vi "AppendObjectNameIfError.vi"(8 "error in (no error)":errorcluster, 10 "GObj Refnum":refnum<vi>, 11 "Control Layout in":refnum<class "Control Layout.lvclass">) -> (0 "error out":errorcluster, 3 "Control Layout out":refnum<class "Control Layout.lvclass">)   [LabVIEW 2010, in "NI_SE_Front Panel Layout.lvlib" / "Control Layout.lvclass"]
uses:
  Control Layout.lvclass
  Object Layout/Object Layout.lvclass
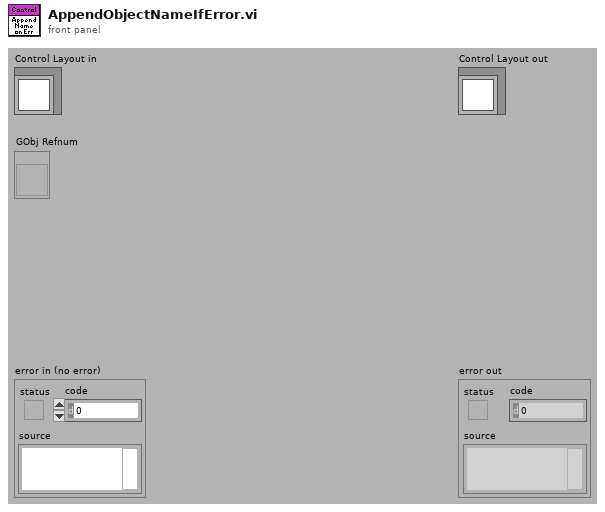
[diagram p1: front panel]
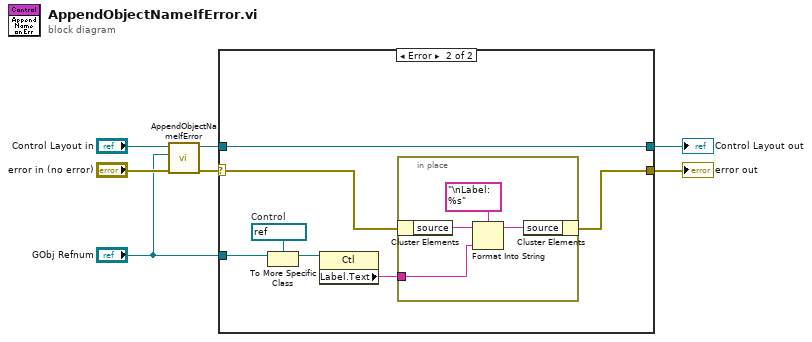
[diagram p0: block diagram]
diagram:
  n1 = call-parent "AppendObjectNameIfError.vi"("error in (no error)"="error in (no error)", "GObj Refnum"="GObj Refnum", "Object Layout in"="Control Layout in") -> ("error out"=w5:errorcluster, "Object Layout out"=w4:refnum<class "Control Layout.lvclass">)  [unwired: 7 in]
  n2 = case shown="Error" w5 {
    selector: w5 -> [w8 w15]
    tunnel: w4 -> [w9 w16]
    tunnel: [w9 w16] -> w3
    tunnel: [w8 w14] -> w2
    tunnel: "GObj Refnum" -> [_ w13]
    frame No Error {
    }
    frame Error {
      w12 = refnum<vi> refnum  # Control
      n3 = To More Specific Class(target class=w12, reference=w13) -> (specific class reference=w11:refnum<vi>)  [unwired: 1 in, 1 out]
      n4 = property class="Ctl"(reference=w11) -> ("Label.Text"=w10:string)  [unwired: 1 in, 2 out]
      n5 = in-place {
        in-place-border: w10 -> [w19]
        n6 = in-place-cluster #1(w15) -> ("source"=w20:string)
        n7 = Format Into String(format string="\nLabel: %s", initial string=w20, w19) -> (resulting string=w17:string)  [unwired: 1 in, 1 out]
        n8 = in-place-cluster #1("source"=w17) -> (w14:errorcluster)
      }
    }
  }
  "error out" <- w2
  "Control Layout out" <- w3
